vi "Utility Parse Flow Rate.vi"(8 "error in (no error)":errorcluster, 11 "String":string) -> (0 "error out":errorcluster, 3 "Numeric":dbl)   [LabVIEW 2020, in "ChromTech Series III Pump.lvlib"]
uses:
  ChromTech Series III Pump.lvlib
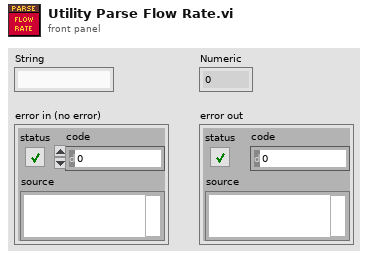
[diagram p1: front panel]
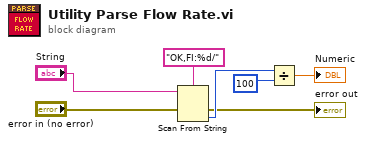
[diagram p0: block diagram]
diagram:
  n1 = Scan From String(format string="OK,FI:%d/", input string="String", error in="error in (no error)") -> (error out=→"error out":errorcluster, output 1=w5:i32)  [unwired: 2 in, 2 out]
  n2 = Divide(x=w5, y=100) -> (x/y=→"Numeric":dbl)
